vi "Read Addr.vi"(8 "error in (no error)":errorcluster, 11 "MKS in":refnum<class "MKS.lvclass">) -> (0 "error out":errorcluster, 2 "Addr":string, 3 "MKS out":refnum<class "MKS.lvclass">)   [LabVIEW 2022 SP3, in "MKS.lvclass"]
uses:
  MKS.lvclass
  MKS.lvclass/MKS.ctl
  Pressure Monitor.lvclass
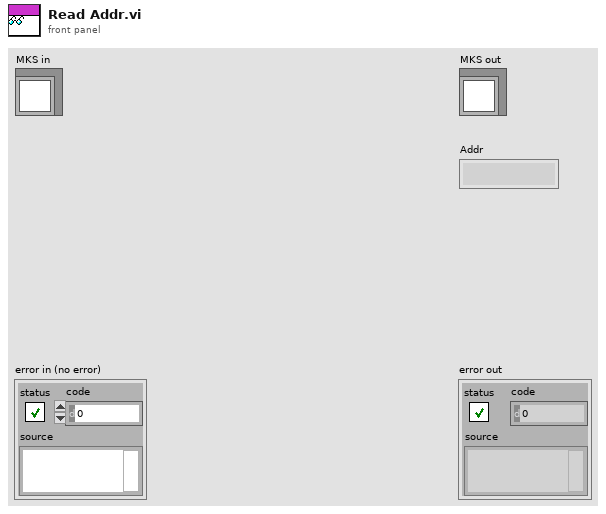
[diagram p1: front panel]
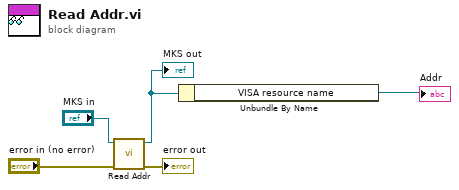
[diagram p0: block diagram]
diagram:
  n1 = call-parent "Read Addr.vi"("error in (no error)"="error in (no error)", "Pressure Monitor in"="MKS in") -> ("error out"=→"error out":errorcluster, "Pressure Monitor out"=w2:refnum<class "MKS.lvclass">)  [unwired: 7 in, 1 out]
  "MKS out" <- w2
  n2 = Unbundle By Name(w2) -> ("VISA resource name"=→"Addr":refnum<visa-resource-name>)
